vi "Shoot.vi"(4 "Time":dbl=1.0, 6 "Speed":dbl=1.0, 11 "error in":errorcluster) -> (3 "error out":errorcluster)   [LabVIEW 2015]
uses:
  References/Refnums.vi
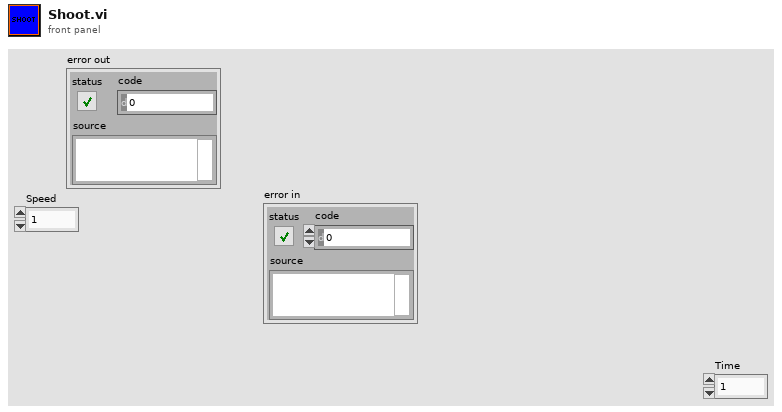
[diagram p1: front panel]
types:
  T1 = typedef "WPI_MotorControlDeviceRef.ctl" = cluster{"DeviceStatus":errorcluster, "Type":T2, "PWM":cluster{"PWM Channel":T3, "DeadBand":T4}, "CAN":cluster{"Device Number":u8, "Control Mode":T5, "Semaphore":T6, "Max Vout":dbl, "TalonSRX Control Mode":T7}, "Invert":bool}
  T2 = typedef "WPI_MotorControlType.ctl" = enum16{"PWM", "CAN", "CANTalonSRX"}
  T3 = typedef "FPGA_DIOPWMChannel.ctl" = enum8{"PWM 0", "PWM 1", "PWM 2", "PWM 3", "PWM 4", "PWM 5", "PWM 6", "PWM 7", "PWM 8", "PWM 9", "PWM MXP 0", "PWM MXP 1", "PWM MXP 2", "PWM MXP 3", "PWM MXP 4", "PWM MXP 5", "PWM MXP 6", "PWM MXP 7", "PWM MXP 8", "PWM MXP 9", "Invalid"}
  T4 = typedef "WPI_PWMDeadband.ctl" = cluster{"Name":string, "maxPositivePwm":i32, "minPositivePwm":i32, "centerPwm":i32, "maxNegativePwm":i32, "minNegativePwm":i32, "angularRange":u16}
  T5 = typedef "WPI_CANJaguar_ControlMode.ctl" = enum8{"Percent VBus", "Current", "Speed", "Position", "Voltage"}
  T6 = typedef "Semaphore RefNum" = refnum<k1>
  T7 = typedef "WPI_CANTalonSRX_APIControlMode.ctl" = enum8{"Percent VBus", "Speed", "Position", "Slave", "Unchanged / Invalid", "Voltage Compensation", "Current", "Motion Profile"}
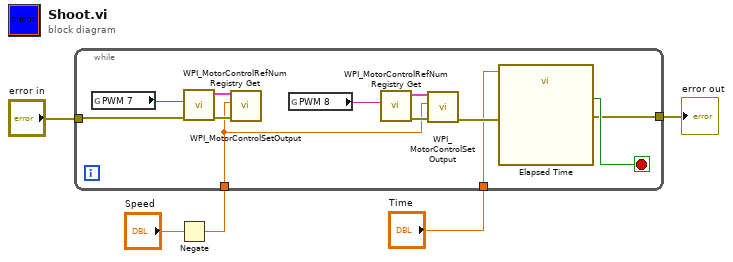
[diagram p0: block diagram]
diagram:
  n1 = Negate(x="Speed") -> (-x=w1:dbl)
  n2 = while {
    tunnel: [w9] -> w5
    tunnel: "error in" -> [w8]
    tunnel: "Time" -> [w7]
    tunnel: w1 -> [w6]
    stop <- w11 stop-if-true
    n3 = global read "Refnums.vi" "PWM 7"() -> (w14:string)
    n4 = call <vilib>:"WPI_MotorControlRefNum Registry Get.vi"("error in (no error)"=w8, "refnum name"=w14) -> ("error out"=w12:errorcluster, "MotorControlDevRef"=w13:T1)  [unwired: 8 in]
    n5 = call <vilib>:"WPI_MotorControlSetOutput.vi"("error in (no error)"=w12, "Output"=w6, "MotorControlDevRef"=w13) -> ()  [unwired: 6 in, 3 out]
    n6 = global read "Refnums.vi" "PWM 8"() -> (w15:string)
    n7 = call <vilib>:"WPI_MotorControlRefNum Registry Get.vi"("refnum name"=w15) -> ("error out"=w17:errorcluster, "MotorControlDevRef"=w16:T1)  [unwired: 9 in]
    n8 = call <vilib>:"WPI_MotorControlSetOutput.vi"("error in (no error)"=w17, "Output"=w6, "MotorControlDevRef"=w16) -> ("error out"=w10:errorcluster)  [unwired: 6 in, 2 out]
    n9 = call "Elapsed Time"("Time Target (s)"=w7, "error in (no error)"=w10) -> ("Time has Elapsed"=w11:bool, "error out"=w9:errorcluster)  [unwired: 10 in, 6 out]
  }
  "error out" <- w5
